vi "Read Attributes.vi"(11 "Send Complete Service Msg":refnum<class "Send Complete Service Msg.lvclass">) -> (2 "Payload":cluster{"Service ID":string})   [LabVIEW 2023, in "Room Service Monitor UI.lvlib" / "Send Complete Service Msg.lvclass"]
uses:
  Send Complete Service Msg.lvclass
  Send Complete Service Msg.lvclass/Send Complete Service Msg.ctl
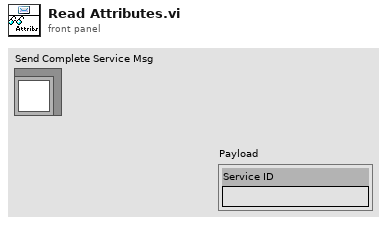
[diagram p1: front panel]
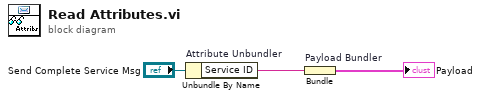
[diagram p0: block diagram]
diagram:
  n1 = Unbundle By Name "Attribute Unbundler"("Send Complete Service Msg") -> ("Service ID"=w1:string)
  n2 = Bundle "Payload Bundler"("Service ID"=w1) -> (→"Payload":cluster{"Service ID":string})  [unwired: 1 in]
